vi "Create Dispatcher.vi"(7 "framework options":T1={"FIFO Options"={"Infinite Timeouts"=FALSE}, "Thread Options"={"Show FP On Call"=FALSE, "Close FP After Call"=FALSE, "Allow Debugging"=FALSE}, "Plugin Options"={"Default Components"=FALSE}, "Performance Options"={"Measure Period"=FALSE, "Measure Rx/Tx Duration"=FALSE}, "Data Server Options"={"Enable Data Server"=FALSE, "Period"=50}} {"Data Server Options"."Period" format="%d ms"}, 8 "error in (no error)":errorcluster, 10 "Plugins":refnum<class "Plugin.lvclass">[](array[class]), 11 "Framework in":refnum<class "Framework.lvclass">) -> (0 "error out":errorcluster, 2 "Dispatcher Thread":refnum<class "Dispatcher Thread.lvclass">, 3 "Framework out":refnum<class "Framework.lvclass">)   [LabVIEW 2021, in "DSF Core.lvlib" / "Framework.lvclass"]
uses:
  Framework.lvclass
  Plugin/Plugin.lvclass
  Thread/Dispatcher/Dispatcher Thread.lvclass
  C:/dev/git/custom-devices/niveristand-data-sharing-framework-custom-device/Source/Core/Classes/Thread/Thread.lvclass
  Framework Options.ctl
  Typedefs/DSF FIFO Options.ctl
  Thread/Thread Options.ctl
  Typedefs/DSF Plugin Options.ctl
  Typedefs/DSF Performance Options.ctl
  Data Server Options.ctl
  Framework.lvclass/Framework.ctl
  Thread/Thread Settings.ctl
  Interface/Interface.lvclass/Interface.ctl
  Thread/Thread.lvclass/Thread.ctl
  Thread/Dispatcher/Dispatcher Thread.lvclass/Dispatcher Thread.ctl
  Plugin/Plugin.lvclass/Plugin.ctl
  Transfer Group/Transfer Group.lvclass/Transfer Group.ctl
  Thread/Set Thread Parameters.vi
  Thread/Set Name.vi
  Thread/Dispatcher/Initialize Plugin Settings.vi
  Interface/New Interface.vi
  Plugin/Get Async Rx Transfer Groups.vi
  Plugin/Get Async Tx Transfer Groups.vi
  Plugin/Get Inline Rx Transfer Groups.vi
  Plugin/Get Inline Tx Transfer Groups.vi
  Transfer Group/Get ID.vi
  Transfer Group/Get Thread.vi
  Plugin/Get Thread Interfaces.vi
  Interface/Create RT FIFO.vi
  Interface/Dispatcher/Dispatcher Interface.lvclass
  C:/dev/git/custom-devices/niveristand-data-sharing-framework-custom-device/Source/Core/Classes/Interface/Interface.lvclass
  Interface/Plugin/Plugin Interface.lvclass
  Thread/Thread.lvclass
  DSF Core.lvlib
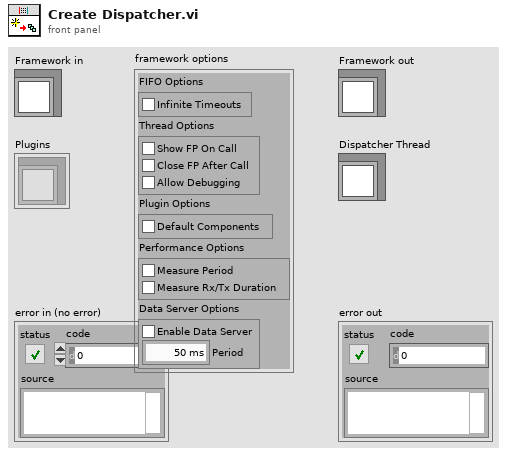
[diagram p1: front panel]
types:
  T1 = typedef "DSF Core.lvlib/Framework.lvclass/Framework Options.ctl" = cluster{"FIFO Options":T2, "Thread Options":T3, "Plugin Options":T4, "Performance Options":T5, "Data Server Options":T6}
  T2 = typedef "DSF Core.lvlib/Framework.lvclass/DSF FIFO Options.ctl" = cluster{"Infinite Timeouts":bool}
  T3 = typedef "DSF Core.lvlib/Thread.lvclass/Thread Options.ctl" = cluster{"Show FP On Call":bool, "Close FP After Call":bool, "Allow Debugging":bool}
  T4 = typedef "DSF Core.lvlib/Framework.lvclass/DSF Plugin Options.ctl" = cluster{"Default Components":bool}
  T5 = typedef "DSF Core.lvlib/DSF Performance Options.ctl" = cluster{"Measure Period":bool, "Measure Rx/Tx Duration":bool}
  T6 = typedef "DSF Core.lvlib/Framework.lvclass/Data Server Options.ctl" = cluster{"Enable Data Server":bool, "Period":u32}
  T7 = typedef "DSF Core.lvlib/Thread.lvclass/Thread Settings.ctl" = cluster{"Priority":u16, "Processor":i32}
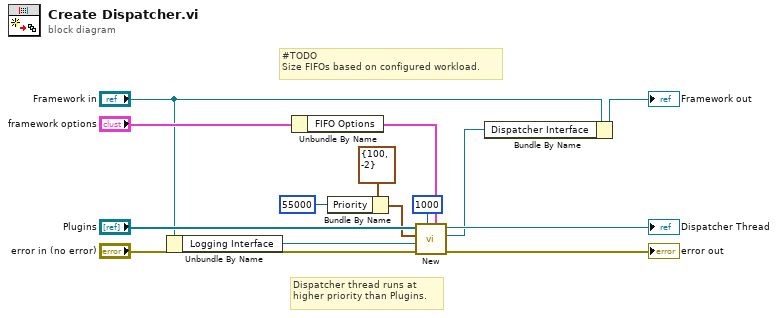
[diagram p0: block diagram]
diagram:
  # "Dispatcher thread runs at higher priority than Plugins."
  # "#TODO\nSize FIFOs based on configured workload."
  n1 = Unbundle By Name("Framework in") -> ("Logging Interface"=w1:refnum<class "Logging Interface.lvclass">)
  n2 = Unbundle By Name("framework options") -> ("FIFO Options"=w3:T2)
  n3 = Bundle By Name(cluster=T7 {"Priority"=100, "Processor"=-2} ("Thread Parameters"), "Priority"=u16 55000 ("priority (100)")) -> (w4:T7)
  n4 = call "New.vi"("FIFO Options"=w3, "fifo depths"=u32 1000, "error in (no error)"="error in (no error)", "Logging Interface"=w1, "Thread Parameters"=w4, "Plugins"="Plugins") -> ("error out"=→"error out":errorcluster, "Dispatcher Interface"=w10:refnum<class "Dispatcher Interface.lvclass">, "Dispatcher Thread"=→"Dispatcher Thread":refnum<class "Dispatcher Thread.lvclass">)  [unwired: 3 in]
  n5 = Bundle By Name(cluster="Framework in", "Dispatcher Interface"=w10) -> (→"Framework out":refnum<class "Framework.lvclass">)
